vi "M9347 Init.vi"(8 "error in (no error)":errorcluster) -> (0 "error out":errorcluster)   [LabVIEW 2023]
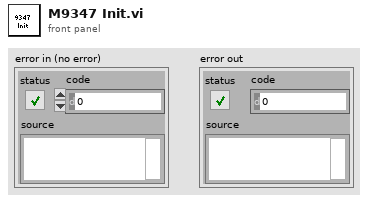
[diagram p1: front panel]
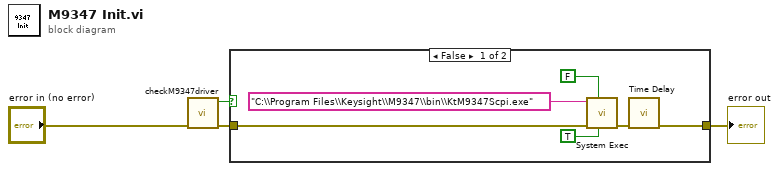
[diagram p0: block diagram]
diagram:
  n1 = call "checkM9347driver.vi"("error in (no error)"="error in (no error)") -> ("error out"=w3:errorcluster, "Checkbox"=w2:bool)  [unwired: 9 in]
  n2 = case shown="False" w2 {
    tunnel: w3 -> [w8 w11]
    tunnel: [w5 w11] -> w1
    frame False {
      n3 = call <vilib>:"System Exec.vi"("run minimized? (F)"=TRUE, "wait until completion? (T)"=FALSE, "error in (no error)"=w8, "command line"="C:\\Program Files\\Keysight\\M9347\\bin\\KtM9347Scpi.exe") -> ("error out"=w6:errorcluster)  [unwired: 4 in, 3 out]
      n4 = call "Time Delay"("error in (no error)"=w6) -> ("error out"=w5:errorcluster)  [unwired: 10 in]
    }
    frame True {
    }
  }
  "error out" <- w1
